vi "GOOP_CheckFileReadonly.vi"(0 "FilePath":path, 11 "error in":errorcluster) -> (4 "IsReadOnly":bool, 15 "error out":errorcluster)   [LabVIEW 2020]
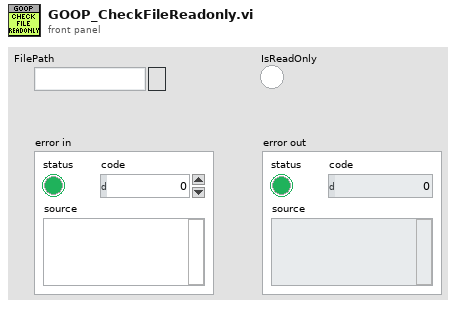
[diagram p1: front panel]
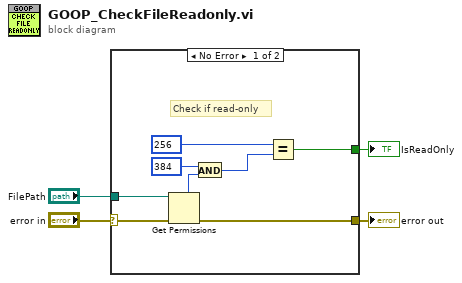
[diagram p0: block diagram]
diagram:
  n1 = case shown="No Error" "error in" {
    selector: "error in" -> [w7 w13]
    tunnel: "FilePath" -> [w8 _]
    tunnel: [w6 w13] -> w2
    tunnel: [w5 _] -> w1
    frame No Error {
      # "Check if read-only"
      n2 = Get Permissions(8:w7, 11:w8) -> (0:w6:errorcluster, 5:w12:i16)  [unwired: 3 out]
      n3 = And(x=i16 384, y=w12) -> (x .and. y?=w10:i16)
      n4 = Equal?(x=i16 256, y=w10) -> (x = y?=w5:bool)
    }
    frame Error {
    }
  }
  "error out" <- w2
  "IsReadOnly" <- w1
